vi "Advance past Number.vi"(7 "JSON":string, 9 "Offset (0)":i32, 11 "Parser State in":T2=enum."Number/Other") -> (1 "Offset past match":i32, 2 "LabVIEW Extension (NaN, Infinity)":bool, 3 "Parser State":T2, 4 "JSON Value Type":T1, 6 "Value start out":i32)   [LabVIEW 2024, in "JSONtext.lvlib"]
uses:
  JSONtext.lvlib
  Parsing State.ctl
  JSON Value Type.ctl
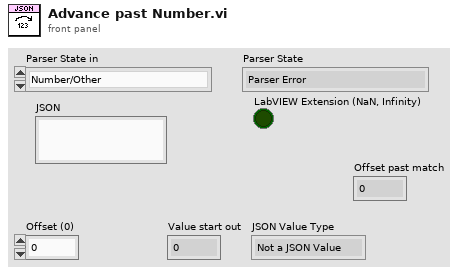
[diagram p1: front panel]
types:
  T1 = typedef "JSONtext.lvlib/JSON Value Type.ctl" = enum16{"Not a JSON Value", "JSON Object", "JSON Array", "String", "Number", "true", "false", "null"}
  T2 = typedef "JSONtext.lvlib/Parsing State.ctl" = enum16{"Parser Error", "Object", "Array", "String", "Number/Other", "Leading Whitespace", "Object end", "Array end", "Value end"}
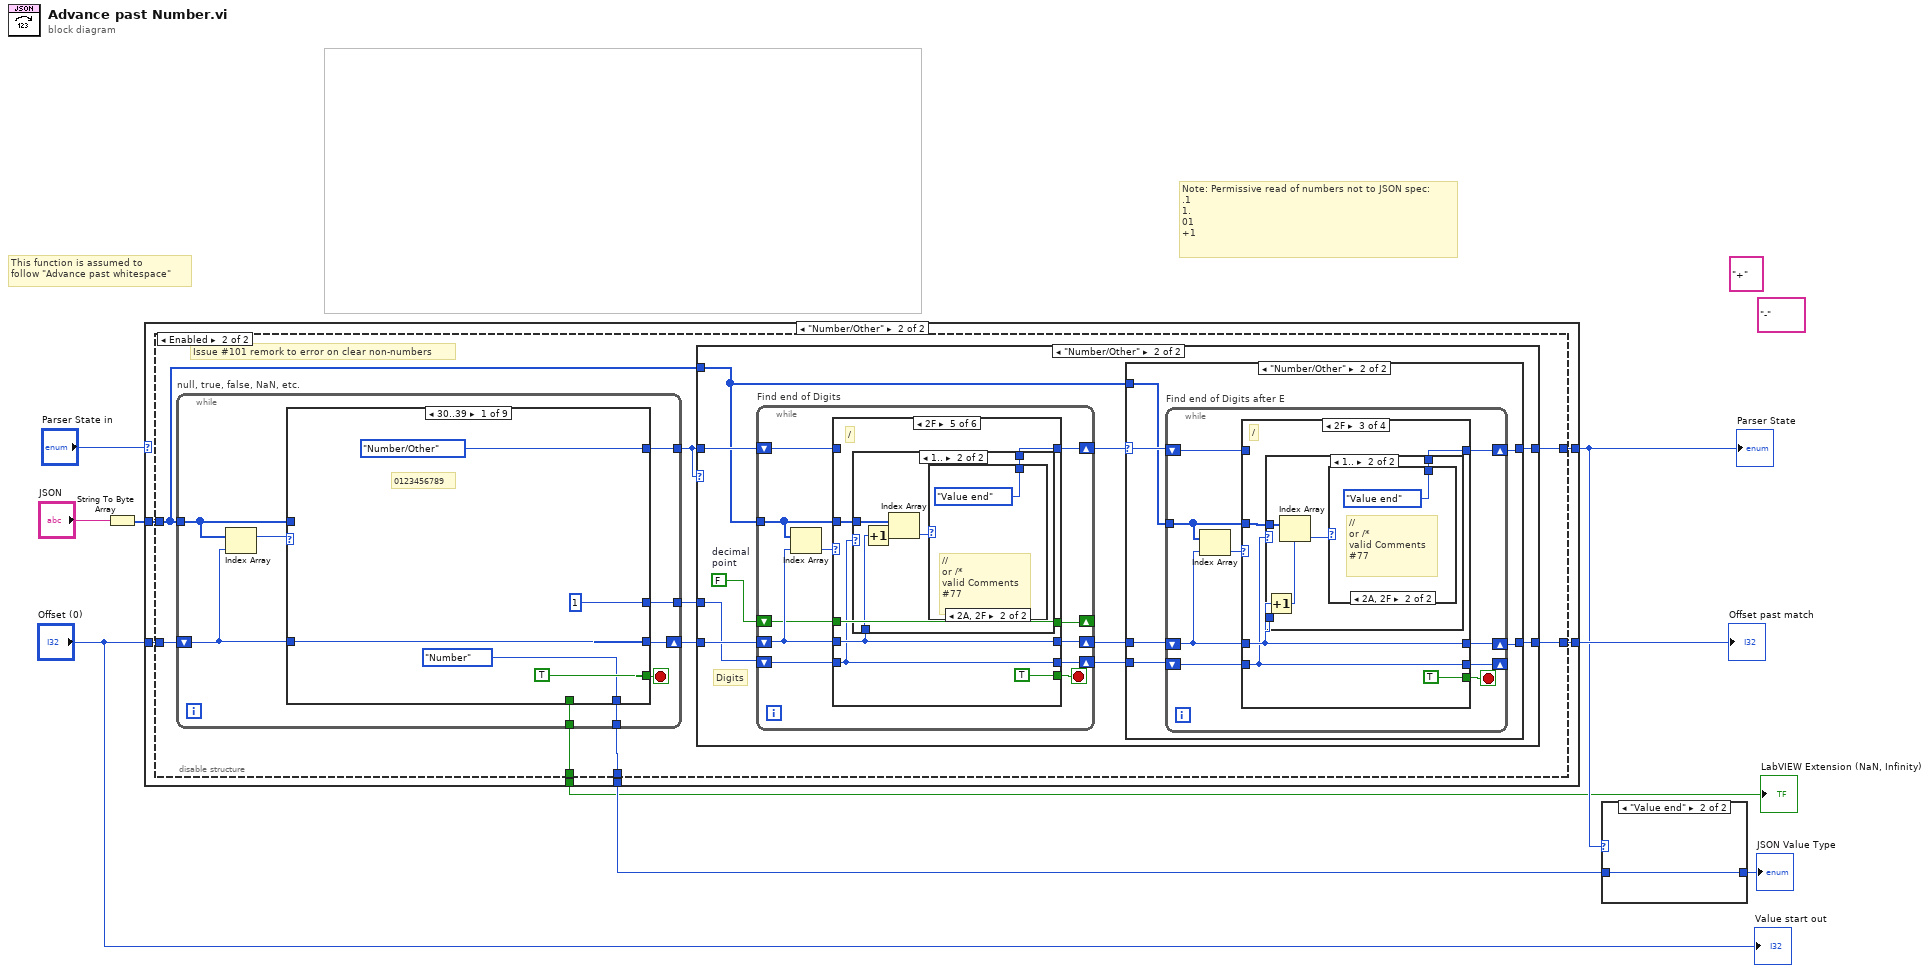
[diagram p0: block diagram]
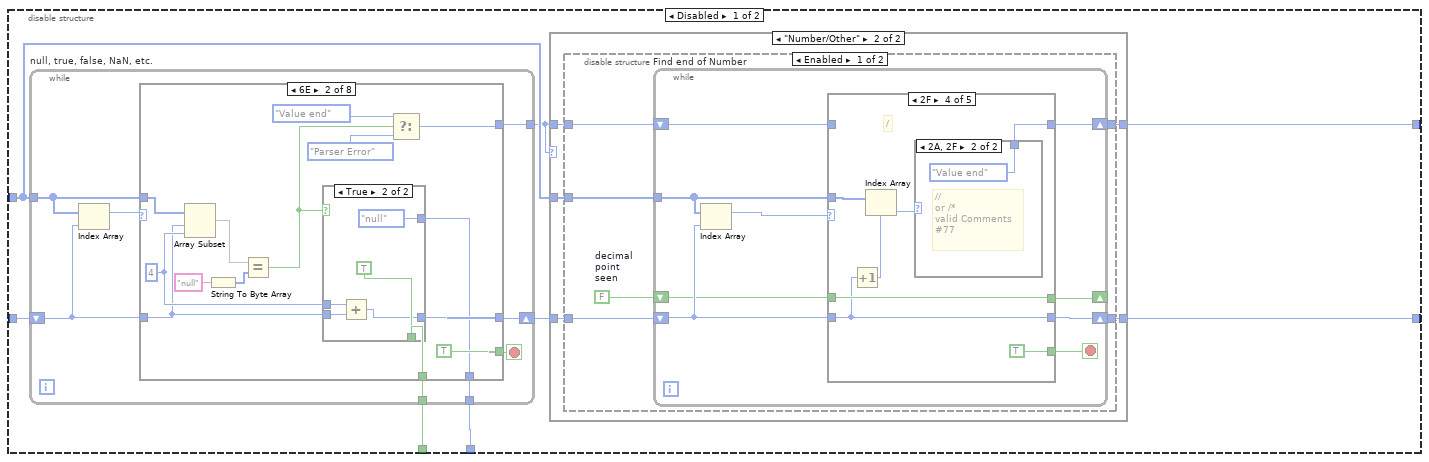
[diagram p3: hidden frame]
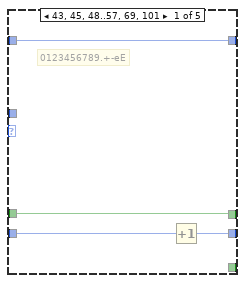
[diagram p5: hidden frame]
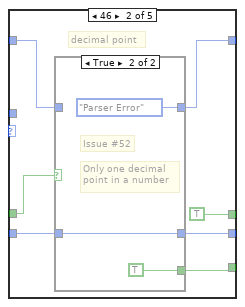
[diagram p6: hidden frame]
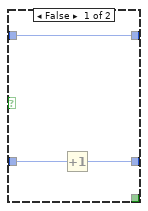
[diagram p7: hidden frame]
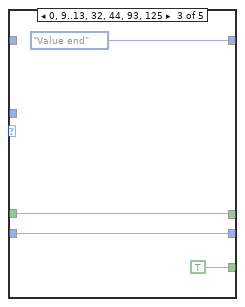
[diagram p8: hidden frame]
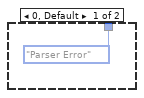
[diagram p9: hidden frame]
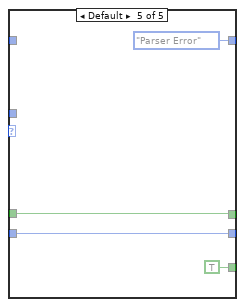
[diagram p10: hidden frame]
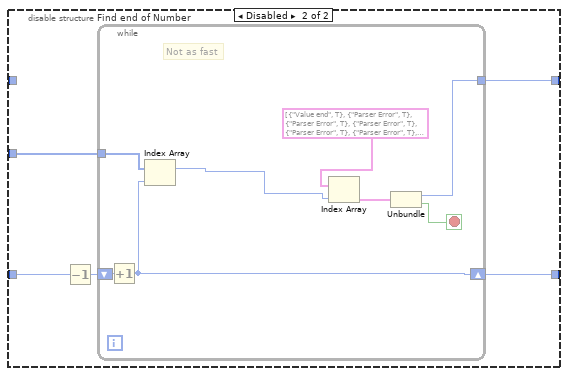
[diagram p11: hidden frame]
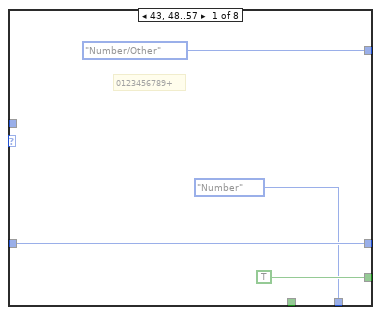
[diagram p12: hidden frame]
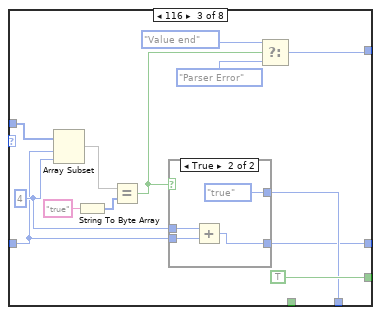
[diagram p14: hidden frame]
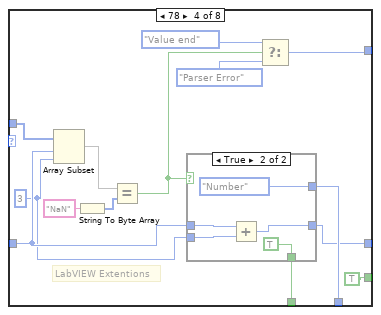
[diagram p16: hidden frame]
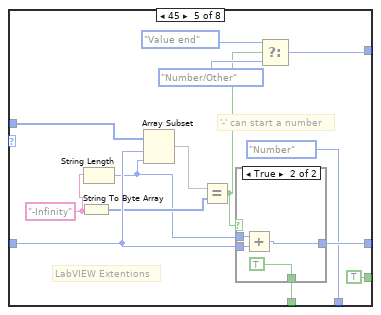
[diagram p18: hidden frame]
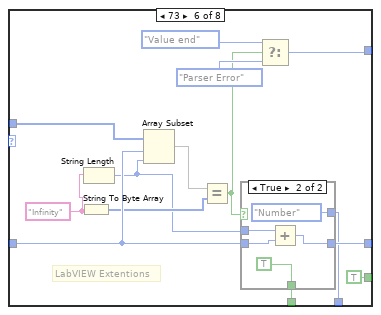
[diagram p20: hidden frame]
diagram:
  (unwired) "+"
  (unwired) "-"
  # "Note: Permissive read of numbers not to JSON spec:\n.1\n1.\n01\n+1"
  # "This function is assumed to \nfollow \"Advance past whitespace\""
  n1 = String To Byte Array(string="JSON") -> (unsigned byte array=w6:u8[])
  n2 = case shown="\"Number/Other\"" "Parser State in" {
    tunnel: [_ w16] -> w4
    tunnel: [w10 w15] -> w9
    tunnel: w6 -> [_ w14]
    tunnel: "Offset (0)" -> [w10 w13]
    tunnel: [_ w12] -> w3
    tunnel: [_ w11] -> w1
    frame "Parser Error", Default {
    }
    frame "Number/Other" {
      n3 = disable-structure shown="Enabled" {
        disable-tunnel: [w24 w229] -> w16
        disable-tunnel: [w23 w228] -> w15
        disable-tunnel: w14 -> [w21 w226]
        disable-tunnel: w13 -> [w19 w224]
        disable-tunnel: [w18 w223] -> w12
        disable-tunnel: [w17 w222] -> w11
        frame Disabled {
          n4 = while "null, true, false, NaN, etc." {
            tunnel: w21 -> [w100]
            shift-right: [w96] -> w22
            shift-left: w19 -> [w97]
            tunnel: [w99] -> w20
            tunnel: [w95] -> w18
            tunnel: [w94] -> w17
            stop <- w98 stop-if-true
            n5 = Index Array(array=w100, index=w97) -> (element=w101:u8)
            n6 = case shown="6E" w101 {
              tunnel: w100 -> [_ w118 w137 w156 w177 w196 w214 _]
              tunnel: [Parsing_State."Number/Other" w115 w134 w153 w175 w194 w211 Parsing_State."Parser Error"] -> w99
              tunnel: [TRUE TRUE TRUE TRUE TRUE TRUE TRUE TRUE] -> w98
              tunnel: w97 -> [w103 w107 w127 w147 w171 w190 w207 w220]
              tunnel: [w103 w106 w126 w145 w170 w189 w205 w220] -> w96
              tunnel: [JSON_Value_Type."Number" w110 w129 w148 JSON_Value_Type."Number" w184 w203 JSON_Value_Type."Not a JSON Value"] -> w95
              tunnel: [_ w109 _ w144 w164 w183 _ _] -> w94
              frame 43, 48..57 {
                # "0123456789+"
              }
              frame 110 {
                w108 = 4 ("length")
                n7 = Array Subset(array=w118, index=w107, length=w108) -> (w116:u8[])
                n8 = String To Byte Array(string="null") -> (unsigned byte array=w117:u8[])
                n9 = Equal?(x=w116, y=w117) -> (x = y?=w111:bool)
                n10 = case shown="True" w111 {
                  tunnel: [_ JSON_Value_Type."null"] -> w110
                  tunnel: [_ TRUE] -> w109
                  tunnel: w108 -> [_ w123]
                  tunnel: w107 -> [w120 w122]
                  tunnel: [w120 w121] -> w106
                  frame False {
                  }
                  frame True {
                    n11 = Add(x=w123, y=w122) -> (x+y=w121:i32)
                  }
                }
                n12 = Select(t=Parsing_State."Value end", s=w111, f=Parsing_State."Parser Error") -> (s? t:f=w115:T2)
              }
              frame 116 {
                w128 = 4 ("length")
                n13 = Array Subset(array=w137, index=w127, length=w128) -> (w135:u8[])
                n14 = String To Byte Array(string="true") -> (unsigned byte array=w136:u8[])
                n15 = Equal?(x=w135, y=w136) -> (x = y?=w130:bool)
                n16 = case shown="True" w130 {
                  tunnel: [_ JSON_Value_Type."true"] -> w129
                  tunnel: w128 -> [_ w142]
                  tunnel: w127 -> [w139 w141]
                  tunnel: [w139 w140] -> w126
                  frame False {
                  }
                  frame True {
                    n17 = Add(x=w142, y=w141) -> (x+y=w140:i32)
                  }
                }
                n18 = Select(t=Parsing_State."Value end", s=w130, f=Parsing_State."Parser Error") -> (s? t:f=w134:T2)
              }
              frame 78 {
                w146 = 3 ("length")
                # "LabVIEW Extentions"
                n19 = Array Subset(array=w156, index=w147, length=w146) -> (w154:u8[])
                n20 = String To Byte Array(string="NaN") -> (unsigned byte array=w155:u8[])
                n21 = Equal?(x=w154, y=w155) -> (x = y?=w149:bool)
                n22 = case shown="True" w149 {
                  tunnel: [_ JSON_Value_Type."Number"] -> w148
                  tunnel: w147 -> [w158 w162]
                  tunnel: w146 -> [_ w161]
                  tunnel: [w158 w160] -> w145
                  tunnel: [_ TRUE] -> w144
                  frame False {
                  }
                  frame True {
                    n23 = Add(x=w162, y=w161) -> (x+y=w160:i32)
                  }
                }
                n24 = Select(t=Parsing_State."Value end", s=w149, f=Parsing_State."Parser Error") -> (s? t:f=w153:T2)
              }
              frame 45 {
                w168 = "-Infinity"
                # "'-' can start a number"
                # "LabVIEW Extentions"
                n25 = String To Byte Array(string=w168) -> (unsigned byte array=w169:u8[])
                n26 = String Length(string=w168) -> (length=w167:i32)
                n27 = Array Subset(array=w177, index=w171, length=w167) -> (w176:u8[])
                n28 = Equal?(x=w176, y=w169) -> (x = y?=w166:bool)
                n29 = case shown="True" w166 {
                  tunnel: w171 -> [w178 w182]
                  tunnel: [w178 w181] -> w170
                  tunnel: w167 -> [_ w180]
                  tunnel: [_ TRUE] -> w164
                  frame False {
                  }
                  frame True {
                    n30 = Add(x=w180, y=w182) -> (x+y=w181:i32)
                  }
                }
                n31 = Select(t=Parsing_State."Value end", s=w166, f=Parsing_State."Number/Other") -> (s? t:f=w175:T2)
              }
              frame 73 {
                w187 = "Infinity"
                # "LabVIEW Extentions"
                n32 = String To Byte Array(string=w187) -> (unsigned byte array=w188:u8[])
                n33 = String Length(string=w187) -> (length=w186:i32)
                n34 = Array Subset(array=w196, index=w190, length=w186) -> (w195:u8[])
                n35 = Equal?(x=w195, y=w188) -> (x = y?=w185:bool)
                n36 = case shown="True" w185 {
                  tunnel: w190 -> [w197 w202]
                  tunnel: [w197 w201] -> w189
                  tunnel: w186 -> [_ w200]
                  tunnel: [_ JSON_Value_Type."Number"] -> w184
                  tunnel: [_ TRUE] -> w183
                  frame False {
                  }
                  frame True {
                    n37 = Add(x=w200, y=w202) -> (x+y=w201:i32)
                  }
                }
                n38 = Select(t=Parsing_State."Value end", s=w185, f=Parsing_State."Parser Error") -> (s? t:f=w194:T2)
              }
              frame 102 {
                w206 = 5 ("length")
                n39 = Array Subset(array=w214, index=w207, length=w206) -> (w212:u8[])
                n40 = String To Byte Array(string="false") -> (unsigned byte array=w213:u8[])
                n41 = Equal?(x=w212, y=w213) -> (x = y?=w204:bool)
                n42 = case shown="True" w204 {
                  tunnel: [_ JSON_Value_Type."false"] -> w203
                  frame False {
                  }
                  frame True {
                  }
                }
                n43 = Add(x=w206, y=w207) -> (x+y=w205:i32)
                n44 = Select(t=Parsing_State."Value end", s=w204, f=Parsing_State."Parser Error") -> (s? t:f=w211:T2)
              }
              frame Default {
              }
            }
          }
          n45 = case shown="\"Number/Other\"" w20 {
            tunnel: [w25 w31] -> w24
            tunnel: [w26 w30] -> w23
            tunnel: w22 -> [w26 w27]
            tunnel: w20 -> [w25 w29]
            tunnel: w21 -> [_ w28]
            frame "Parser Error", Default {
            }
            frame "Number/Other" {
              n46 = disable-structure shown="Enabled" {
                disable-tunnel: [w37 w85] -> w31
                disable-tunnel: [w36 w84] -> w30
                disable-tunnel: w29 -> [w35 _]
                disable-tunnel: w28 -> [w34 w83]
                disable-tunnel: w27 -> [w33 w82]
                frame Enabled {
                  w32 = FALSE  # decimal point seen
                  n47 = while "Find end of Number" {
                    tunnel: w34 -> [w46]
                    shift-right: [w42] -> w36
                    shift-left: w33 -> [w40]
                    shift-right: [w44] -> w37
                    shift-left: w35 -> [w45]
                    shift-right: [w39] -> _
                    shift-left: w32 -> [w38]
                    stop <- w43 stop-if-true
                    n48 = Index Array(array=w46, index=w40) -> (element=w41:u8)
                    n49 = case shown="2F" w41 {
                      tunnel: w46 -> [_ _ _ w70 _]
                      tunnel: w45 -> [w50 w53 _ _ _]
                      tunnel: [w50 w52 Parsing_State."Value end" w68 Parsing_State."Parser Error"] -> w44
                      tunnel: [_ w51 TRUE TRUE TRUE] -> w43
                      tunnel: w40 -> [w49 w57 w65 w72 w80]
                      tunnel: [w48 w56 w65 w72 w80] -> w42
                      tunnel: [w47 TRUE w64 w73 w77] -> w39
                      tunnel: w38 -> [w47 w54 w64 w73 w77]
                      frame 43, 45, 48..57, 69, 101 {
                        # "0123456789.+-eE"
                        n50 = Increment(x=w49) -> (x+1=w48:i32)
                      }
                      frame 46 {
                        # "decimal point"
                        n51 = case shown="True" w54 {
                          tunnel: w57 -> [w60 w62]
                          tunnel: [w59 w62] -> w56
                          tunnel: [w58 Parsing_State."Parser Error"] -> w52
                          tunnel: w53 -> [w58 _]
                          tunnel: [_ TRUE] -> w51
                          frame False {
                            n52 = Increment(x=w60) -> (x+1=w59:i32)
                          }
                          frame True {
                            # "Only one decimal\npoint in a number"
                            # "Issue #52"
                          }
                        }
                      }
                      frame 0, 9..13, 32, 44, 93, 125 {
                      }
                      frame 47 {
                        # "/"
                        n53 = Increment(x=w72) -> (x+1=w71:i32)
                        n54 = Index Array(array=w70, index=w71) -> (element=w69:u8)
                        n55 = case shown="2A, 2F" w69 {
                          tunnel: [Parsing_State."Parser Error" Parsing_State."Value end"] -> w68
                          frame 0, Default {
                          }
                          frame 42, 47 {
                            # "//\nor /*\nvalid Comments\n#77"
                          }
                        }
                      }
                      frame Default {
                      }
                    }
                  }
                }
                frame Disabled {
                  n56 = Decrement(x=w82) -> (x-1=w81:i32)
                  n57 = while "Find end of Number" {
                    tunnel: w83 -> [w93]
                    shift-right: [w86] -> w84
                    shift-left: w81 -> [w92]
                    tunnel: [w87] -> w85
                    stop <- w88 stop-if-true
                    # "Not as fast"
                    n58 = Increment(x=w92) -> (x+1=w86:i32)
                    n59 = Index Array(array=w93, index=w86) -> (element=w89:u8)
                    n60 = Index Array(array=cluster{T2, bool}[] [{enum."Value end", TRUE}, {enum."Parser Error", TRUE}, {enum."Parser Error", TRUE}, {enum."Parser Error", TRUE}, {enum."Parser Error", TRUE}, {enum."Parser Error", TRUE}, {enum."Parser Error", TRUE}, {enum."Parser Error", TRUE}, {enum."Parser Error", TRUE}, {enum."Value end", TRUE}, {enum."Value end", TRUE}, {enum."Value end", TRUE}, {enum."Value end", TRUE}, {enum."Value end", TRUE}, {enum."Parser Error", TRUE}, {enum."Parser Error", TRUE}, {enum."Parser Error", TRUE}, {enum."Parser Error", TRUE}, {enum."Parser Error", TRUE}, {enum."Parser Error", TRUE}, {enum."Parser Error", TRUE}, {enum."Parser Error", TRUE}, {enum."Parser Error", TRUE}, {enum."Parser Error", TRUE}, {enum."Parser Error", TRUE}, {enum."Parser Error", TRUE}, {enum."Parser Error", TRUE}, {enum."Parser Error", TRUE}, {enum."Parser Error", TRUE}, {enum."Parser Error", TRUE}, {enum."Parser Error", TRUE}, {enum."Parser Error", TRUE}, {enum."Value end", TRUE}, {enum."Parser Error", TRUE}, {enum."Parser Error", TRUE}, {enum."Parser Error", TRUE}, {enum."Parser Error", TRUE}, {enum."Parser Error", TRUE}, {enum."Parser Error", TRUE}, {enum."Parser Error", TRUE}, {enum."Parser Error", TRUE}, {enum."Parser Error", TRUE}, {enum."Parser Error", TRUE}, {enum."Number/Other", FALSE}, {enum."Value end", TRUE}, {enum."Number/Other", FALSE}, {enum."Number/Other", FALSE}, {enum."Parser Error", TRUE}, {enum."Number/Other", FALSE}, {enum."Number/Other", FALSE}, {enum."Number/Other", FALSE}, {enum."Number/Other", FALSE}, {enum."Number/Other", FALSE}, {enum."Number/Other", FALSE}, {enum."Number/Other", FALSE}, {enum."Number/Other", FALSE}, {enum."Number/Other", FALSE}, {enum."Number/Other", FALSE}, {enum."Parser Error", TRUE}, {enum."Parser Error", TRUE}, {enum."Parser Error", TRUE}, {enum."Parser Error", TRUE}, {enum."Parser Error", TRUE}, {enum."Parser Error", TRUE}, {enum."Parser Error", TRUE}, {enum."Parser Error", TRUE}, {enum."Parser Error", TRUE}, {enum."Parser Error", TRUE}, {enum."Parser Error", TRUE}, {enum."Number/Other", FALSE}, {enum."Parser Error", TRUE}, {enum."Parser Error", TRUE}, {enum."Parser Error", TRUE}, {enum."Parser Error", TRUE}, {enum."Parser Error", TRUE}, {enum."Parser Error", TRUE}, {enum."Parser Error", TRUE}, {enum."Parser Error", TRUE}, {enum."Parser Error", TRUE}, {enum."Parser Error", TRUE}, {enum."Parser Error", TRUE}, {enum."Parser Error", TRUE}, {enum."Parser Error", TRUE}, {enum."Parser Error", TRUE}, {enum."Parser Error", TRUE}, {enum."Parser Error", TRUE}, {enum."Parser Error", TRUE}, {enum."Parser Error", TRUE}, {enum."Parser Error", TRUE}, {enum."Parser Error", TRUE}, {enum."Parser Error", TRUE}, {enum."Parser Error", TRUE}, {enum."Parser Error", TRUE}, {enum."Value end", TRUE}, {enum."Parser Error", TRUE}, {enum."Parser Error", TRUE}, {enum."Parser Error", TRUE}, {enum."Parser Error", TRUE}, {enum."Parser Error", TRUE}, {enum."Parser Error", TRUE}, {enum."Parser Error", TRUE}, {enum."Number/Other", FALSE}, {enum."Parser Error", TRUE}, {enum."Parser Error", TRUE}, {enum."Parser Error", TRUE}, {enum."Parser Error", TRUE}, {enum."Parser Error", TRUE}, {enum."Parser Error", TRUE}, {enum."Parser Error", TRUE}, {enum."Parser Error", TRUE}, {enum."Parser Error", TRUE}, {enum."Parser Error", TRUE}, {enum."Parser Error", TRUE}, {enum."Parser Error", TRUE}, {enum."Parser Error", TRUE}, {enum."Parser Error", TRUE}, {enum."Parser Error", TRUE}, {enum."Parser Error", TRUE}, {enum."Parser Error", TRUE}, {enum."Parser Error", TRUE}, {enum."Parser Error", TRUE}, {enum."Parser Error", TRUE}, {enum."Parser Error", TRUE}, {enum."Parser Error", TRUE}, {enum."Parser Error", TRUE}, {enum."Value end", TRUE}] ("Array"), index=w89) -> (element=w90:cluster{T2, bool})
                    n61 = Unbundle(w90) -> (w87:T2, w88:bool)
                  }
                }
              }
            }
          }
        }
        frame Enabled {
          # "Issue #101 remork to error on clear non-numbers"
          n62 = while "null, true, false, NaN, etc." {
            tunnel: w226 -> [w369]
            shift-right: [w365] -> w227
            shift-left: w224 -> [w366]
            tunnel: [w368] -> w225
            tunnel: [w364] -> w223
            tunnel: [w363] -> w222
            tunnel: [w362] -> w221
            stop <- w367 stop-if-true
            n63 = Index Array(array=w369, index=w366) -> (element=w370:u8)
            n64 = case shown="30..39" w370 {
              tunnel: w369 -> [_ _ w393 w412 w431 w452 w472 w490 _]
              tunnel: [Parsing_State."Number/Other" Parsing_State."Number/Other" w390 w409 w428 w450 w470 w487 Parsing_State."Parser Error"] -> w368
              tunnel: [TRUE TRUE TRUE TRUE TRUE TRUE TRUE TRUE TRUE] -> w367
              tunnel: w366 -> [w373 w378 w382 w402 w422 w446 w466 w483 w496]
              tunnel: [w373 w376 w381 w401 w420 w445 w465 w481 w496] -> w365
              tunnel: [JSON_Value_Type."Number" JSON_Value_Type."Number" w385 w404 w423 JSON_Value_Type."Number" w460 w479 JSON_Value_Type."Not a JSON Value"] -> w364
              tunnel: [_ _ w384 _ w419 w439 w459 _ _] -> w363
              tunnel: [1 _ _ _ _ _ _ _ _] -> w362
              frame 48..57 {
                # "0123456789"
              }
              frame 43 {
                # "+"
                n65 = Increment(x=w378) -> (x+1=w376:i32)
              }
              frame 110 {
                w383 = 4 ("length")
                n66 = Array Subset(array=w393, index=w382, length=w383) -> (w391:u8[])
                n67 = String To Byte Array(string="null") -> (unsigned byte array=w392:u8[])
                n68 = Equal?(x=w391, y=w392) -> (x = y?=w386:bool)
                n69 = case shown="True" w386 {
                  tunnel: [_ JSON_Value_Type."null"] -> w385
                  tunnel: [_ TRUE] -> w384
                  tunnel: w383 -> [_ w398]
                  tunnel: w382 -> [w395 w397]
                  tunnel: [w395 w396] -> w381
                  frame False {
                  }
                  frame True {
                    n70 = Add(x=w398, y=w397) -> (x+y=w396:i32)
                  }
                }
                n71 = Select(t=Parsing_State."Value end", s=w386, f=Parsing_State."Parser Error") -> (s? t:f=w390:T2)
              }
              frame 116 {
                w403 = 4 ("length")
                n72 = Array Subset(array=w412, index=w402, length=w403) -> (w410:u8[])
                n73 = String To Byte Array(string="true") -> (unsigned byte array=w411:u8[])
                n74 = Equal?(x=w410, y=w411) -> (x = y?=w405:bool)
                n75 = case shown="True" w405 {
                  tunnel: [_ JSON_Value_Type."true"] -> w404
                  tunnel: w403 -> [_ w417]
                  tunnel: w402 -> [w414 w416]
                  tunnel: [w414 w415] -> w401
                  frame False {
                  }
                  frame True {
                    n76 = Add(x=w417, y=w416) -> (x+y=w415:i32)
                  }
                }
                n77 = Select(t=Parsing_State."Value end", s=w405, f=Parsing_State."Parser Error") -> (s? t:f=w409:T2)
              }
              frame 78 {
                w421 = 3 ("length")
                # "LabVIEW Extentions"
                n78 = Array Subset(array=w431, index=w422, length=w421) -> (w429:u8[])
                n79 = String To Byte Array(string="NaN") -> (unsigned byte array=w430:u8[])
                n80 = Equal?(x=w429, y=w430) -> (x = y?=w424:bool)
                n81 = case shown="True" w424 {
                  tunnel: [_ JSON_Value_Type."Number"] -> w423
                  tunnel: w422 -> [w433 w437]
                  tunnel: w421 -> [_ w436]
                  tunnel: [w433 w435] -> w420
                  tunnel: [_ TRUE] -> w419
                  frame False {
                  }
                  frame True {
                    n82 = Add(x=w437, y=w436) -> (x+y=w435:i32)
                  }
                }
                n83 = Select(t=Parsing_State."Value end", s=w424, f=Parsing_State."Parser Error") -> (s? t:f=w428:T2)
              }
              frame 45 {
                w443 = "-Infinity"
                # "'-' can start a number"
                # "LabVIEW Extentions"
                n84 = String To Byte Array(string=w443) -> (unsigned byte array=w444:u8[])
                n85 = String Length(string=w443) -> (length=w442:i32)
                n86 = Array Subset(array=w452, index=w446, length=w442) -> (w451:u8[])
                n87 = Equal?(x=w451, y=w444) -> (x = y?=w441:bool)
                n88 = case shown="False" w441 {
                  tunnel: w446 -> [w454 w458]
                  tunnel: [w453 w457] -> w445
                  tunnel: w442 -> [_ w456]
                  tunnel: [_ TRUE] -> w439
                  frame False {
                    n89 = Increment(x=w454) -> (x+1=w453:i32)
                  }
                  frame True {
                    n90 = Add(x=w456, y=w458) -> (x+y=w457:i32)
                  }
                }
                n91 = Select(t=Parsing_State."Value end", s=w441, f=Parsing_State."Number/Other") -> (s? t:f=w450:T2)
              }
              frame 73 {
                w463 = "Infinity"
                # "LabVIEW Extentions"
                n92 = String To Byte Array(string=w463) -> (unsigned byte array=w464:u8[])
                n93 = String Length(string=w463) -> (length=w462:i32)
                n94 = Array Subset(array=w472, index=w466, length=w462) -> (w471:u8[])
                n95 = Equal?(x=w471, y=w464) -> (x = y?=w461:bool)
                n96 = case shown="True" w461 {
                  tunnel: w466 -> [w473 w478]
                  tunnel: [w473 w477] -> w465
                  tunnel: w462 -> [_ w476]
                  tunnel: [_ JSON_Value_Type."Number"] -> w460
                  tunnel: [_ TRUE] -> w459
                  frame False {
                  }
                  frame True {
                    n97 = Add(x=w476, y=w478) -> (x+y=w477:i32)
                  }
                }
                n98 = Select(t=Parsing_State."Value end", s=w461, f=Parsing_State."Parser Error") -> (s? t:f=w470:T2)
              }
              frame 102 {
                w482 = 5 ("length")
                n99 = Array Subset(array=w490, index=w483, length=w482) -> (w488:u8[])
                n100 = String To Byte Array(string="false") -> (unsigned byte array=w489:u8[])
                n101 = Equal?(x=w488, y=w489) -> (x = y?=w480:bool)
                n102 = case shown="True" w480 {
                  tunnel: [_ JSON_Value_Type."false"] -> w479
                  frame False {
                  }
                  frame True {
                  }
                }
                n103 = Add(x=w482, y=w483) -> (x+y=w481:i32)
                n104 = Select(t=Parsing_State."Value end", s=w480, f=Parsing_State."Parser Error") -> (s? t:f=w487:T2)
              }
              frame Default {
              }
            }
          }
          n105 = case shown="\"Number/Other\"" w225 {
            tunnel: [w230 w236] -> w229
            tunnel: [w231 w235] -> w228
            tunnel: w227 -> [w231 w240]
            tunnel: w225 -> [w230 w241]
            tunnel: w226 -> [_ w233]
            tunnel: w221 -> [_ w238]
            frame "Parser Error", Default {
            }
            frame "Number/Other" {
              w239 = FALSE  # decimal point
              # "Digits"
              n106 = while "Find end of Digits" {
                tunnel: w233 -> [w297]
                shift-right: [w293] -> w234
                shift-left: w240 -> [w291]
                shift-right: [w295] -> w237
                shift-left: w241 -> [w296]
                shift-right: [w290] -> _
                shift-left: w239 -> [w289]
                shift-right: [w288] -> w232
                shift-left: w238 -> [w287]
                stop <- w294 stop-if-true
                n107 = Index Array(array=w297, index=w291) -> (element=w292:u8)
                n108 = case shown="2F" w292 {
                  tunnel: w297 -> [_ w308 _ _ w345 _]
                  tunnel: w296 -> [w303 _ w325 _ _ _]
                  tunnel: [w303 w309 w324 w337 w344 Parsing_State."Parser Error"] -> w295
                  tunnel: [_ w311 w323 TRUE TRUE TRUE] -> w294
                  tunnel: w291 -> [w302 w313 w329 w339 w346 w361]
                  tunnel: [w301 w305 w328 w339 w346 w361] -> w293
                  tunnel: [w300 w312 TRUE w338 w347 w358] -> w290
                  tunnel: w289 -> [w300 w312 w326 w338 w347 w358]
                  tunnel: [w298 w306 w322 w336 w343 w357] -> w288
                  tunnel: w287 -> [w299 w310 w322 w336 w343 w357]
                  frame 48..57 {
                    # "0123456789"
                    n109 = Increment(x=w299) -> (x+1=w298:i32)
                    n110 = Increment(x=w302) -> (x+1=w301:i32)
                  }
                  frame 69, 101 {
                    w311 = TRUE  # E
                    # "eE"
                    n111 = Increment(x=w313) -> (x+1=w304:i32)
                    n112 = case "Had digits before E?" shown="1.." w310 {
                      tunnel: [Parsing_State."Parser Error" Parsing_State."Number/Other"] -> w309
                      frame ..0 {
                      }
                      frame 1.. {
                      }
                    }
                    n113 = Index Array(array=w308, index=w304) -> (element=w307:u8)
                    n114 = case shown="2B, 2D" w307 {
                      tunnel: [_ _ 1] -> w306
                      tunnel: [w314 w315 w317] -> w305
                      tunnel: w304 -> [w314 w316 w318]
                      frame Default {
                      }
                      frame 43, 45 {
                        # "+-"
                        n115 = Increment(x=w316) -> (x+1=w315:i32)
                      }
                      frame 48..57 {
                        # "0123456789"
                        n116 = Increment(x=w318) -> (x+1=w317:i32)
                      }
                    }
                  }
                  frame 46 {
                    # "decimal point"
                    n117 = case shown="True" w326 {
                      tunnel: w329 -> [w332 w334]
                      tunnel: [w331 w334] -> w328
                      tunnel: [w330 Parsing_State."Parser Error"] -> w324
                      tunnel: w325 -> [w330 _]
                      tunnel: [_ TRUE] -> w323
                      frame False {
                        n118 = Increment(x=w332) -> (x+1=w331:i32)
                      }
                      frame True {
                        # "Only one decimal\npoint in a number"
                        # "Issue #52"
                      }
                    }
                  }
                  frame 0, 9..13, 32, 44, 93, 125 {
                    n119 = case "Had digits" shown="1.." w336 {
                      tunnel: [Parsing_State."Parser Error" Parsing_State."Value end"] -> w337
                      frame ..0 {
                      }
                      frame 1.. {
                      }
                    }
                  }
                  frame 47 {
                    # "/"
                    n120 = case shown="1.." w343 {
                      tunnel: w346 -> [_ w354]
                      tunnel: w345 -> [_ w352]
                      tunnel: [Parsing_State."Parser Error" w350] -> w344
                      frame 0, Default {
                        # "No Digits"
                      }
                      frame 1.. {
                        n121 = Increment(x=w354) -> (x+1=w353:i32)
                        n122 = Index Array(array=w352, index=w353) -> (element=w351:u8)
                        n123 = case shown="2A, 2F" w351 {
                          tunnel: [Parsing_State."Parser Error" Parsing_State."Value end"] -> w350
                          frame 0, Default {
                          }
                          frame 42, 47 {
                            # "//\nor /*\nvalid Comments\n#77"
                          }
                        }
                      }
                    }
                  }
                  frame Default {
                  }
                }
              }
              n124 = case shown="\"Number/Other\"" w237 {
                selector: w237 -> [w243 w248]
                tunnel: [w243 w247] -> w236
                tunnel: [w242 w249] -> w235
                tunnel: w234 -> [w242 w245]
                tunnel: w233 -> [_ w246]
                tunnel: w232 -> [_ w244]
                frame "Parser Error", Default {
                }
                frame "Number/Other" {
                  n125 = while "Find end of Digits after E" {
                    tunnel: w246 -> [w258]
                    shift-right: [w254] -> w249
                    shift-left: w245 -> [w252]
                    shift-right: [w256] -> w247
                    shift-left: w248 -> [w257]
                    shift-right: [w251] -> _
                    shift-left: w244 -> [w250]
                    stop <- w255 stop-if-true
                    n126 = Index Array(array=w258, index=w252) -> (element=w253:u8)
                    n127 = case shown="2F" w253 {
                      tunnel: w258 -> [_ _ w273 _]
                      tunnel: w257 -> [w263 _ _ _]
                      tunnel: [w263 w265 w272 Parsing_State."Parser Error"] -> w256
                      tunnel: [_ TRUE TRUE TRUE] -> w255
                      tunnel: w252 -> [w262 w266 w271 w286]
                      tunnel: [w261 w266 w271 w286] -> w254
                      tunnel: [w259 w264 w270 w283] -> w251
                      tunnel: w250 -> [w260 w264 w270 w283]
                      frame 48..57 {
                        # "0123456789"
                        n128 = Increment(x=w260) -> (x+1=w259:i32)
                        n129 = Increment(x=w262) -> (x+1=w261:i32)
                      }
                      frame 0, 9..13, 32, 44, 93, 125 {
                        n130 = case "Had digits" shown="1.." w264 {
                          tunnel: [Parsing_State."Parser Error" Parsing_State."Value end"] -> w265
                          frame ..0 {
                          }
                          frame 1.. {
                          }
                        }
                      }
                      frame 47 {
                        # "/"
                        n131 = case shown="1.." w270 {
                          tunnel: w271 -> [_ w280]
                          tunnel: w273 -> [_ w278]
                          tunnel: [Parsing_State."Parser Error" w276] -> w272
                          frame 0, Default {
                            # "No Digits"
                          }
                          frame 1.. {
                            n132 = Increment(x=w280) -> (x+1=w279:i32)
                            n133 = Index Array(array=w278, index=w279) -> (element=w277:u8)
                            n134 = case shown="2A, 2F" w277 {
                              tunnel: [Parsing_State."Parser Error" Parsing_State."Value end"] -> w276
                              frame 0, Default {
                              }
                              frame 42, 47 {
                                # "//\nor /*\nvalid Comments\n#77"
                              }
                            }
                          }
                        }
                      }
                      frame Default {
                      }
                    }
                  }
                }
              }
            }
          }
        }
      }
    }
  }
  "Parser State" <- w4
  "Offset past match" <- w9
  "LabVIEW Extension (NaN, Infinity)" <- w1
  n135 = case shown="\"Value end\"" w4 {
    tunnel: w3 -> [_ w498]
    tunnel: [JSON_Value_Type."Not a JSON Value" w498] -> w2
    frame "Parser Error", Default {
    }
    frame "Value end" {
    }
  }
  "JSON Value Type" <- w2
  "Value start out" <- "Offset (0)"
